vi "Benchmark Class call.vi"() -> ()   [LabVIEW 2016]
uses:
  Math.lvclass
panel:
  out "us/iteration":dbl format="%.6f"
  in  "iterations":i32=1000000000
  # "0.079540 us/iteration 1E9 iterations"
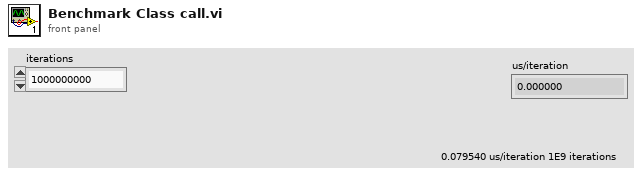
[diagram p1: front panel]
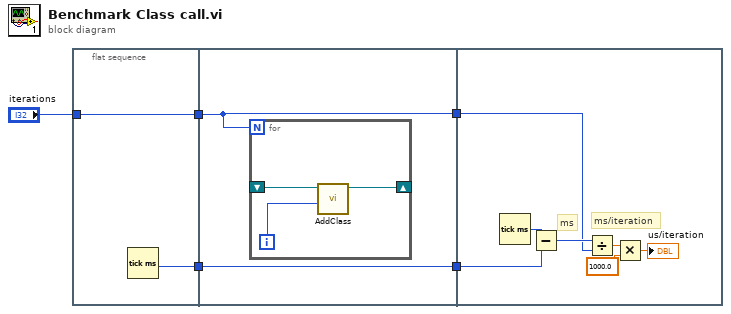
[diagram p0: block diagram]
diagram:
  n1 = flat-sequence {
    tunnel: [w7] -> w5
    tunnel: "iterations" -> [w6]
    tunnel: [w6] -> w1
    tunnel: w5 -> [w9]
    tunnel: [w9] -> w4
    tunnel: [w8] -> w3
    tunnel: w1 -> [w8]
    tunnel: w4 -> [w13]
    tunnel: w3 -> [w14]
    frame #0 {
      n2 = Tick Count (ms)() -> (millisecond timer value=w7:u32)
    }
    frame #1 {
      n3 = for {
        N: w8 -> [_]
        shift-right: [w10] -> _
        shift-left: _ -> [w11]
        i -> [w12]
        n4 = call "AddClass.vi"("Count"=w12, "Math.lvclass"=w11) -> ("Math.lvclass out"=w10:refnum<class "Math.lvclass">)  [unwired: 9 in]
      }
    }
    frame #2 {
      # "ms/iteration"
      # "ms"
      n5 = Tick Count (ms)() -> (millisecond timer value=w19:u32)
      n6 = Subtract(x=w19, y=w13) -> (x-y=w18:u32)
      n7 = Divide(x=w18, y=w14) -> (x/y=w17:dbl)
      n8 = Multiply(x=w17, y=1000.0) -> (x*y=→"us/iteration":dbl)
    }
  }
